vi "RT Main.vi"() -> ()   [LabVIEW 2016]
doc: "The top-level VI for the RIO Eval Kit.\n\nThis VI runs through multiple stages. Each stage demonstrates different features of the RIO Eval Kit. The program uses a \"Queued Message Handler\" architecture. The top loop reads and writes information to and from the FPGA. That information is sent to the bottom through a queue. The information being transfered includes both the data and the type of message being sent. The bottom loop then handles displaying the appropriate information on the LCD."
uses:
  controls/SystemStates.ctl
  <vilib>/EmbeddedDisplay/Hitachi HD44780/Common/Control/screen size.ctl
  <vilib>/EmbeddedDisplay/Hitachi HD44780/Common/Control/font configuration.ctl
  controls/Queue Data.ctl
  controls/SoundOptions.ctl
  <vilib>/TagLibrary/Create Tag (Double).vi
  <vilib>/TagLibrary/Create Tag (Int).vi
  <vilib>/FPGAPlugInAG/sbRIO-9637/niLvFpga_Open_sbRIO-9637.vi
  <vilib>/rvi/interface/common/dynamic/niFpgaDynamicAddResources.vi
  <vilib>/Utility/error.llb/Error Cluster From Error Code.vi
  <vilib>/rvi/errors/niLvFpgaAdjustHostInterfaceError.vi
  <vilib>/measure/mascope.llb/Amplitude and Levels 1 chan.vi
  <vilib>/TagLibrary/Write (Int).vi
  <vilib>/TagLibrary/Write (Double).vi
  <vilib>/FPGAPlugInAG/Dynamic/niLvFpga_Close_Dynamic.vi
  <vilib>/rvi/interface/nirviOpenFPGA/nirviOpenFPGA.xnode
  FPGA Bitfiles/LabVIEWRIOEvalua_FPGATarget_FPGA_fRdPegB0rcM.lvbitx
  <vilib>/rvi/interface/nirviMethod/nirviMethod.xnode
  <vilib>/rvi/interface/nirviReadWriteControl/nirviReadWriteControl.xnode
  <vilib>/rvi/interface/nirviCloseFPGA/nirviCloseFPGA.xnode
  <vilib>/EmbeddedDisplay/Hitachi HD44780/Host/HD44780 Host.lvlib
  <vilib>/EmbeddedDisplay/Hitachi HD44780/Common/HD44780 Common.lvlib
  NiFpgaLv.dll
  <vilib>/rvi/interface/Simulation/niFpgaSimulationCallBeginRW.vi
  <vilib>/measure/NI_MAPro.lvlib
  <vilib>/FPGAPlugInAG/Dynamic/niLvFpga_ReadFifo_Dynamic.vi
  <vilib>/rvi/errors/niLvFpgaMergeErrorWithErrorCode.vi
  <vilib>/TagLibrary/TagLibrary.lvlib
  <resource>/objmgr/niTag.rc
panel:
  out "Signal":dbl[](graph)
  out "Alarm":bool
  in  "Alarm Threshold":dbl=4.0
  out "Amplitude":dbl format="%#_3g"
  # "Start by turning encoder right to kickoff first stage, and \ncontinue turning right to complete all three stages. Stop \nthe program at any time by pressing the right button (PB2)."
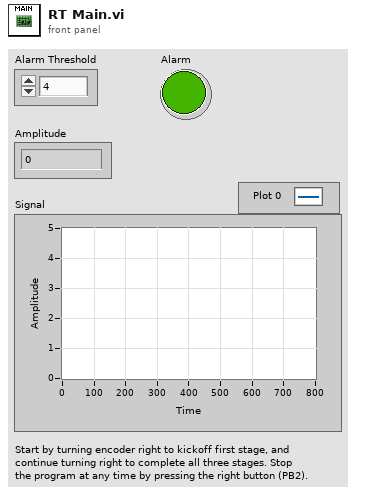
[diagram p1: front panel]
types:
  T1 = typedef "Queue Data.ctl" = cluster{"Current Pos > Threshold?":bool, "Current Pos > Previous?":bool, "Amplitude":dbl, "Stage Number":string}
  T2 = typedef "HD44780 Common.lvlib/font configuration.ctl" = enum8{"5x8 & 2 lines", "5x10 & 1 line", "5x8 & 1 line"}
  T3 = typedef "HD44780 Common.lvlib/screen size.ctl" = enum8{"8x1", "8x2", "12x4", "16x1", "16x2", "16x4", "20x1", "20x2", "20x4", "24x1", "24x2", "40x2", "40x4"}
  T4 = typedef "SystemStates.ctl" = enum16{"Shutdown", "Stage 1", "Stage 2", "Stage 3", "Alarm State"}
  T5 = typedef "SoundOptions.ctl" = enum16{"Ding", "Boing", "Buzzer", "Horn"}
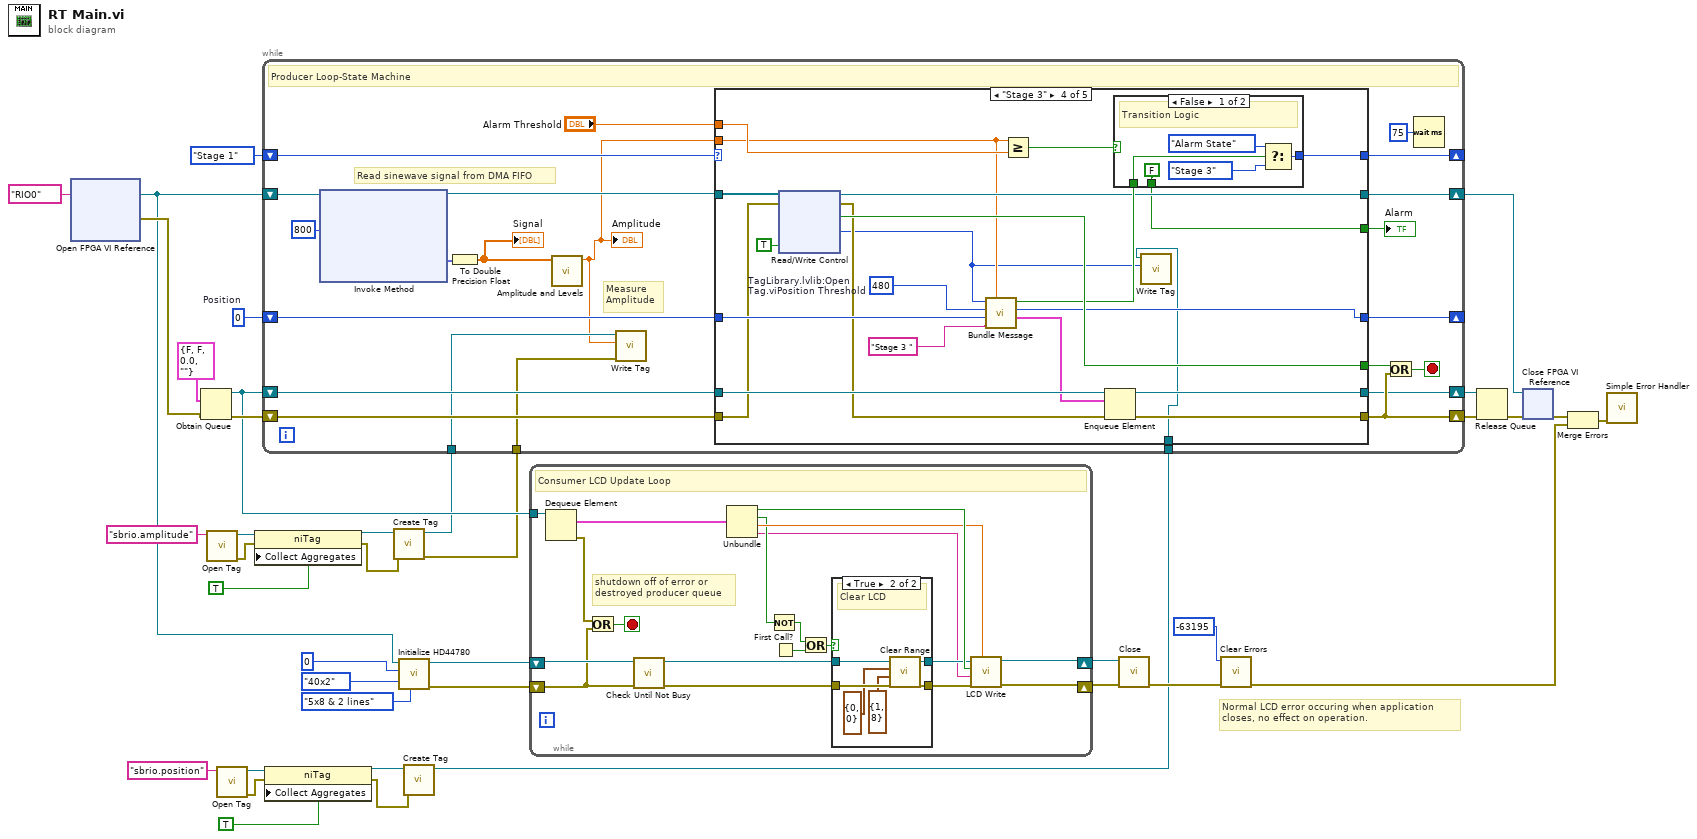
[diagram p0: block diagram]
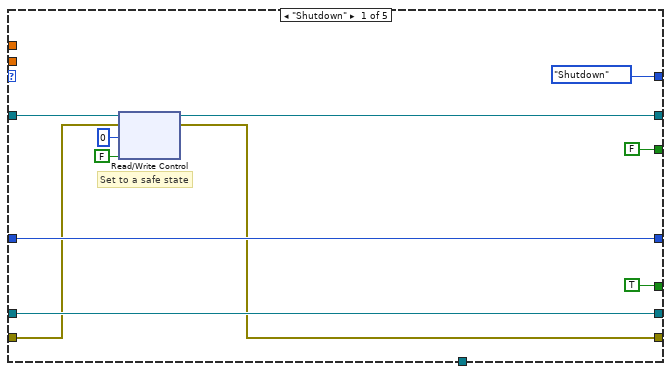
[diagram p3: hidden frame]
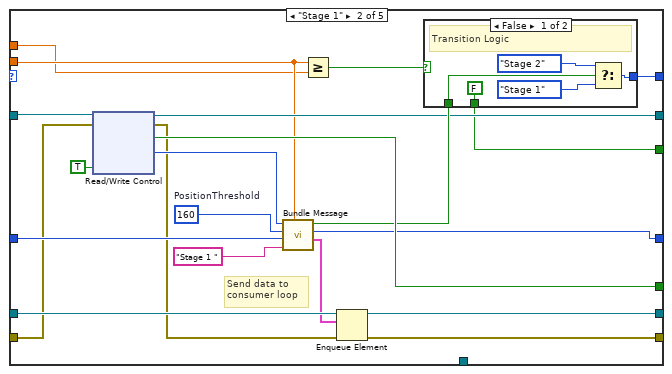
[diagram p4: hidden frame]
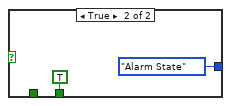
[diagram p5: hidden frame]
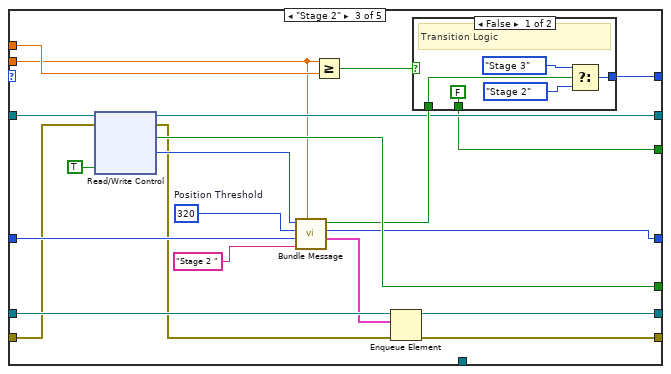
[diagram p6: hidden frame]
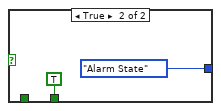
[diagram p7: hidden frame]
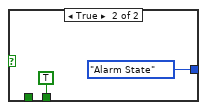
[diagram p8: hidden frame]
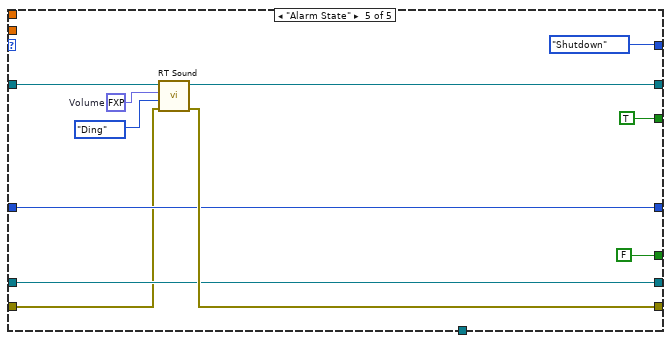
[diagram p9: hidden frame]
diagram:
  w19 = i16 0  # Position
  # "Normal LCD error occuring when application\ncloses, no effect on operation."
  n1 = xnode "Open FPGA VI Reference"("resource name"=tag "RIO0") -> ("FPGA VI Reference Out"=w21:refnum<k20>, "error out"=w25:errorcluster)  [unwired: 1 in]
  n2 = Obtain Queue(element data type=T1 {"Current Pos > Threshold?"=FALSE, "Current Pos > Previous?"=FALSE, "Amplitude"=0.0, "Stage Number"=""} ("output to queue"), error in (no error)=w25) -> (queue out=w22:refnum<queue>, error out=w24:errorcluster)  [unwired: 3 in, 1 out]
  n3 = call <vilib>:"Open Tag.vi"("tag path"="sbrio.amplitude") -> ("error out"=w10:errorcluster, "tag reference out"=w13:refnum<k21>)  [unwired: 9 in]
  n4 = call <vilib>:"Open Tag.vi"("tag path"="sbrio.position") -> ("error out"=w6:errorcluster, "tag reference out"=w4:refnum<k21>)  [unwired: 9 in]
  n5 = property class="niTag"(reference=w13, error in=w10, "Collect Aggregates"=TRUE) -> (reference out=w12:refnum<k21>, error out=w11:errorcluster)
  n6 = property class="niTag"(reference=w4, error in=w6, "Collect Aggregates"=TRUE) -> (reference out=w1:refnum<k21>, error out=w5:errorcluster)
  n7 = call-poly <vilib>:"Create Tag.vi"("error in (no error)"=w11, "tag reference in"=w12) -> ("error out"=w8:errorcluster, "tag reference out"=w15:refnum<k21>)  [unwired: 8 in]
  n8 = call <vilib>:"Initialize HD44780.vi"("font configuration (5x8 & 2 lines)"=font_configuration."5x8 & 2 lines", "screen size"=screen_size."40x2", "device index"=i8 0, "FPGA VI Reference in"=w21) -> ("error out"=w31:errorcluster, "LCD out"=w32:refnum<class "Character LCD.lvclass">)  [unwired: 6 in]
  n9 = call-poly <vilib>:"Create Tag.vi"("error in (no error)"=w5, "tag reference in"=w1) -> ("tag reference out"=w2:refnum<k21>)  [unwired: 8 in, 1 out]
  n10 = while {
    shift-right: [w56] -> w38
    shift-left: w24 -> [w45]
    shift-right: [w54] -> w39
    shift-left: w22 -> [w62]
    shift-right: [w58] -> _
    shift-left: SystemStates."Stage 1" ("Enum") -> [w59]
    shift-right: [w46] -> _
    shift-left: w19 -> [w57]
    shift-right: [w53] -> w20
    shift-left: w21 -> [w51]
    tunnel: w15 -> [w44]
    tunnel: w8 -> [w43]
    tunnel: w2 -> [w42]
    stop <- w60 stop-if-true
    # "Measure\nAmplitude"
    # "Read sinewave signal from DMA FIFO"
    # "Producer Loop-State Machine"
    n11 = xnode "Invoke Method"("FPGA VI Reference In"=w51, "Number of Elements"=u32 800) -> ("FPGA VI Reference Out"=w49:refnum<k20>, "Data"=w52:fxp<+/-,24,5>[])  [unwired: 2 in, 2 out]
    n12 = To Double Precision Float(number=w52) -> (double precision float=w41:dbl[])
    "Signal" <- w41
    n13 = call-poly <vilib>:"Amplitude and Levels.vi"("signal in"=w41) -> ("amplitude"=w40:dbl)  [unwired: 7 in, 3 out]
    "Amplitude" <- w40
    n14 = call-poly <vilib>:"Write Tag.vi"("error in (no error)"=w43, "double"=w40, "tag reference in"=w44) -> ()  [unwired: 7 in, 2 out]
    n15 = case shown="\"Stage 3\"" w59 {
      tunnel: w62 -> [w66 w94 w122 w151 w165]
      tunnel: [w65 w93 w121 w150 w169] -> w56
      tunnel: [TRUE w92 w120 w149 FALSE ("E-Stop")] -> w55
      tunnel: [SystemStates."Shutdown" ("Enum") w91 w119 w148 SystemStates."Shutdown" ("Enum")] -> w58
      tunnel: w57 -> [w67 w78 w106 w136 w161]
      tunnel: [w66 w85 w113 w143 w165] -> w54
      tunnel: w49 -> [w70 w84 w112 w142 w160]
      tunnel: [w69 w83 w111 w141 w164] -> w53
      tunnel: w40 -> [_ w80 w109 w139 _]
      tunnel: [FALSE w81 w107 w137 TRUE] -> w48
      tunnel: "Alarm Threshold" -> [_ w79 w110 w140 _]
      tunnel: [w67 w77 w105 w135 w161] -> w46
      tunnel: w45 -> [w64 w74 w102 w132 w159]
      tunnel: w42 -> [_ _ _ w130 _]
      frame "Shutdown" {
        # "Set to a safe state"
        n16 = xnode "Read/Write Control"("FPGA VI Reference In"=w70, "error in"=w64, "Position"=i16 0, "PWM"=FALSE) -> ("FPGA VI Reference Out"=w69:refnum<k20>, "error out"=w65:errorcluster)
      }
      frame "Stage 1" {
        w87 = i16 160  # PositionThreshold
        # "Send data to\nconsumer loop"
        n17 = xnode "Read/Write Control"("FPGA VI Reference In"=w84, "error in"=w74, "PWM"=TRUE) -> ("FPGA VI Reference Out"=w83:refnum<k20>, "error out"=w75:errorcluster, "E-Stop"=w92:bool, "Position"=w86:i16)
        n18 = call "Bundle Message.vi"("Amplitude"=w80, "Stage Number"="Stage 1 " ("text"), "Previous Position"=w78, "Position Threshold"=w87, "Current Position"=w86) -> ("Output to queue"=w76:T1, "Output Position"=w77:i16, "Transition?"=w89:bool)  [unwired: 4 in]
        n19 = Greater Or Equal?(x=w80, y=w79) -> (x >= y?=w82:bool)
        n20 = Enqueue Element(queue=w94, element=w76, error in (no error)=w75) -> (queue out=w85:refnum<queue>, error out=w93:errorcluster)  [unwired: 1 in, 1 out]
        n21 = case shown="False" w82 {
          tunnel: [w97 SystemStates."Alarm State" ("Enum")] -> w91
          tunnel: w89 -> [w96 _]
          tunnel: [FALSE TRUE] -> w81
          frame False {
            # "Transition Logic"
            n22 = Select(t=SystemStates."Stage 2" ("Enum"), s=w96, f=SystemStates."Stage 1" ("Enum")) -> (s? t:f=w97:T4)
          }
          frame True {
          }
        }
      }
      frame "Stage 2" {
        w115 = i16 320  # Position Threshold
        n23 = xnode "Read/Write Control"("FPGA VI Reference In"=w112, "error in"=w102, "PWM"=TRUE) -> ("FPGA VI Reference Out"=w111:refnum<k20>, "error out"=w103:errorcluster, "E-Stop"=w120:bool, "Position"=w114:i16)
        n24 = call "Bundle Message.vi"("Amplitude"=w109, "Stage Number"="Stage 2 " ("text"), "Previous Position"=w106, "Position Threshold"=w115, "Current Position"=w114) -> ("Output to queue"=w104:T1, "Output Position"=w105:i16, "Transition?"=w116:bool)  [unwired: 4 in]
        n25 = Greater Or Equal?(x=w109, y=w110) -> (x >= y?=w108:bool)
        n26 = Enqueue Element(queue=w122, element=w104, error in (no error)=w103) -> (queue out=w113:refnum<queue>, error out=w121:errorcluster)  [unwired: 1 in, 1 out]
        n27 = case shown="False" w108 {
          tunnel: [w125 SystemStates."Alarm State" ("Enum")] -> w119
          tunnel: w116 -> [w124 _]
          tunnel: [FALSE TRUE] -> w107
          frame False {
            # "Transition Logic"
            n28 = Select(t=SystemStates."Stage 3" ("Enum"), s=w124, f=SystemStates."Stage 2" ("Enum")) -> (s? t:f=w125:T4)
          }
          frame True {
          }
        }
      }
      frame "Stage 3" {
        w144 = i16 480  # TagLibrary.lvlib:Open Tag.viPosition Threshold
        n29 = xnode "Read/Write Control"("FPGA VI Reference In"=w142, "error in"=w132, "PWM"=TRUE) -> ("FPGA VI Reference Out"=w141:refnum<k20>, "error out"=w133:errorcluster, "E-Stop"=w149:bool, "Position"=w131:i16)
        n30 = call "Bundle Message.vi"("Amplitude"=w139, "Stage Number"="Stage 3 " ("text"), "Previous Position"=w136, "Position Threshold"=w144, "Current Position"=w131) -> ("Output to queue"=w134:T1, "Output Position"=w135:i16, "Transition?"=w145:bool)  [unwired: 4 in]
        n31 = Greater Or Equal?(x=w139, y=w140) -> (x >= y?=w138:bool)
        n32 = Enqueue Element(queue=w151, element=w134, error in (no error)=w133) -> (queue out=w143:refnum<queue>, error out=w150:errorcluster)  [unwired: 1 in, 1 out]
        n33 = case shown="False" w138 {
          tunnel: [w154 SystemStates."Alarm State" ("Enum")] -> w148
          tunnel: w145 -> [w153 _]
          tunnel: [FALSE TRUE] -> w137
          frame False {
            # "Transition Logic"
            n34 = Select(t=SystemStates."Alarm State" ("Enum"), s=w153, f=SystemStates."Stage 3" ("Enum")) -> (s? t:f=w154:T4)
          }
          frame True {
          }
        }
        n35 = call-poly <vilib>:"Write Tag.vi"("int"=w131, "tag reference in"=w130) -> ()  [unwired: 8 in, 2 out]
      }
      frame "Alarm State" {
        w167 = fxp<+/-,32,16> 5.0  # Volume
        n36 = call "RT Sound.vi"("error in"=w159, "Sound Options"=SoundOptions."Ding" ("Enum"), "Volume"=w167, "FPGA VI Reference In"=w160) -> ("error out"=w169:errorcluster, "FPGA VI Reference Out"=w164:refnum<k20>)  [unwired: 6 in]
      }
    }
    "Alarm" <- w48
    n37 = Or(x=w55, y=w56) -> (x .or. y?=w60:bool)
    n38 = Wait (ms)(milliseconds to wait=u32 75) -> ()  [unwired: 1 out]
  }
  n39 = while {
    shift-right: [w172] -> w30
    shift-left: w32 -> [w188]
    shift-right: [w171] -> w29
    shift-left: w31 -> [w187]
    tunnel: w22 -> [w186]
    stop <- w180 stop-if-true
    # "shutdown off of error or \ndestroyed producer queue"
    # "Consumer LCD Update Loop"
    n40 = Dequeue Element(queue=w186) -> (element=w183:T1, error out=w184:errorcluster)  [unwired: 2 in, 2 out]
    n41 = Or(x=w184, y=w187) -> (x .or. y?=w180:bool)
    n42 = call "Check Until Not Busy.vi"("error in"=w187, "LCD in"=w188) -> ("error out"=w181:errorcluster, "LCD out"=w182:refnum<class "Character LCD.lvclass">)  [unwired: 8 in]
    n43 = Unbundle(w183) -> ("Current Pos > Threshold?"=w185:bool, "Current Pos > Previous?"=w176:bool, "Amplitude"=w179:dbl, "Stage Number"=w170:string)
    n44 = Not(x=w176) -> (.not. x?=w173:bool)
    n45 = First Call?() -> (First Call?: T/F=w174:bool)
    n46 = Or(x=w173, y=w174) -> (x .or. y?=w175:bool)
    n47 = case shown="True" w175 {
      tunnel: w182 -> [w190 w196]
      tunnel: w181 -> [w189 w195]
      tunnel: [w189 w194] -> w177
      tunnel: [w190 w193] -> w178
      frame False {
      }
      frame True {
        # "Clear LCD"
        n48 = call <vilib>:"Clear Range.vi"("error in (no error)"=w195, "end position (end of line)"=cluster{"row":i8, "column":i8} {"row"=1, "column"=8} ("start position"), "start position"=cluster{"row":i8, "column":i8} {"row"=0, "column"=0}, "LCD in"=w196) -> ("error out"=w194:errorcluster, "LCD out"=w193:refnum<class "Character LCD.lvclass">)  [unwired: 6 in]
      }
    }
    n49 = call "LCD Write.vi"("Amplitude"=w179, "error in (no error)"=w177, "Stage Number"=w170, "Current Pos > Threshold?"=w185, "Character LCD in"=w178) -> ("error out"=w171:errorcluster, "LCD out"=w172:refnum<class "Character LCD.lvclass">)  [unwired: 4 in]
  }
  n50 = call <vilib>:"Close.vi"("error in (no error)"=w29, "LCD in"=w30) -> ("error out"=w16:errorcluster)  [unwired: 9 in]
  n51 = call <vilib>:"Clear Errors.vi"("error in (no error)"=w16, "specific error code to clear (0: all)"=-63195) -> ("error out"=w18:errorcluster)  [unwired: 4 in, 1 out]
  n52 = Release Queue(queue=w39, error in (no error)=w38) -> (error out=w37:errorcluster)  [unwired: 1 in, 2 out]
  n53 = xnode "Close FPGA VI Reference"("FPGA VI Reference In"=w20, "error in"=w37) -> ("error out"=w36:errorcluster)
  n54 = Merge Errors(w36, w18) -> (w28:errorcluster)
  n55 = call <vilib>:"Simple Error Handler.vi"("error in (no error)"=w28) -> ()  [unwired: 4 in, 5 out]
